vi "Close.vi"(8 "error in (no error)":errorcluster {"code" format="%.0x"}, 11 "instrument handle":refnum<k15>) -> (0 "error out":errorcluster {"code" format="%.0x"})   [LabVIEW 2020, in "Keysight DAQ970.lvlib"]
doc: "Closes the I/O session to the instrument. Driver methods and properties that access the instrument are not accessible after Close is called."
uses:
  Keysight DAQ970.lvlib
  KtDAQ970.dll
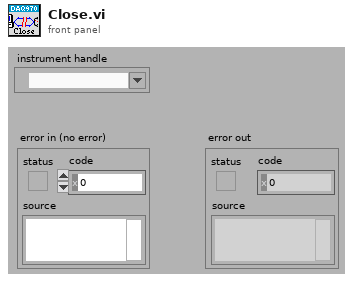
[diagram p1: front panel]
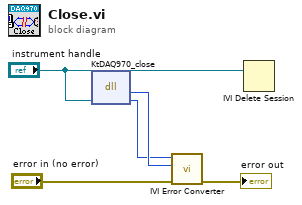
[diagram p0: block diagram]
diagram:
  n1 = dll-call lib="KtDAQ970**.dll" fn="KtDAQ970_close" ("LabVIEW:Ivi_CloseAndGetError")("session"="instrument handle") -> ("return type"=w2:i32, "session"=w1:u32)  [unwired: 3 in, 2 out]
  n2 = call "IVI Error Converter.vi"("error in (no error)"="error in (no error)", "IVI error code (0)"=w2, "instrument handle"=w1) -> ("error out"=→"error out":errorcluster)  [unwired: 7 in, 1 out]
  n3 = IVI Delete Session(11:"instrument handle") -> ()
